vi "Commands to ITX.vi"(1 "Commands":string) -> (0 "ITX Commands":string)   [LabVIEW 2019, in "LV-Data.ITX.lvclass"]
uses:
  LV-Data.ITX.lvclass
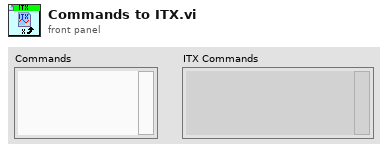
[diagram p1: front panel]
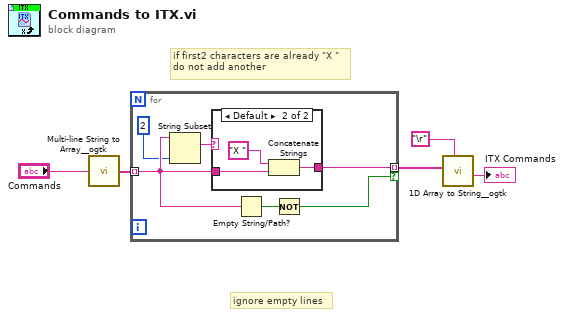
[diagram p0: block diagram]
diagram:
  # "ignore empty lines"
  # "if first2 characters are already \"X \"\ndo not add another"
  n1 = call <userlib>:"Multi-line String to Array__ogtk.vi"("string"="Commands") -> ("lines"=w3:string[])
  n2 = for {
    tunnel: w3 -> [w8] mode=indexing
    tunnel: [w11] -> w2 mode=indexing if=w9
    n3 = String Subset(string=w8, length (rest)=2 ("length (rest)")) -> (substring=w7:string)  [unwired: 1 in]
    n4 = case shown="Default" w7 {
      tunnel: [w12 w15] -> w11
      tunnel: w8 -> [w12 w13]
      frame "X " {
      }
      frame Default {
        n5 = Concatenate Strings("X " ("string"), w13) -> (w15:string)
      }
    }
    n6 = Empty String/Path?(string/path=w8) -> (empty?=w10:bool)
    n7 = Not(x=w10) -> (.not. x?=w9:bool)
  }
  n8 = call <userlib>:"1D Array to String__ogtk.vi"("delimiter (Tab)"="\r", "Array of Strings"=w2) -> ("delimited string"=→"ITX Commands":string)  [unwired: 9 in]
